vi "Zad1-2.vi"() -> ()   [LabVIEW 2015]
panel:
  in  "Losowanie":bool
  out "Numeric":dbl
  # "Losuj"
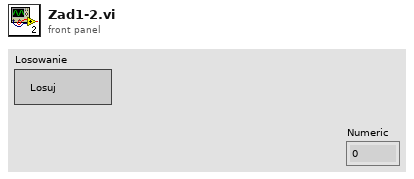
[diagram p1: front panel]
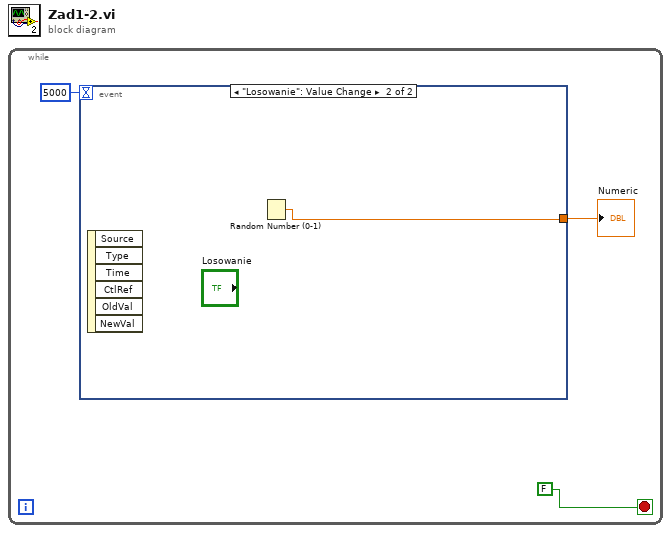
[diagram p0: block diagram]
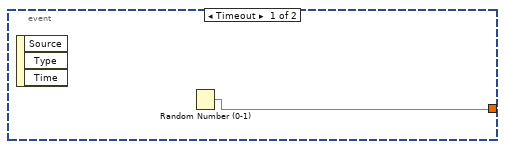
[diagram p2: hidden frame]
diagram:
  n1 = while {
    stop <- FALSE stop-if-true
    n2 = event shown="[1] \"Losowanie\": Value Change" {
      selector: _ -> [_ _]
      dyn-events: _ -> [_ _]
      timeout: 5000 -> [_ _]
      tunnel: [w4 w5] -> w1
      event Timeout {
        n3 = event-data() -> ()  [unwired: 1 in, 3 out]
        n4 = Random Number (0-1)() -> (number: 0 to 1=w4:dbl)
      }
      event "Losowanie": Value Change {
        n5 = event-data() -> ()  [unwired: 1 in, 6 out]
        n6 = Random Number (0-1)() -> (number: 0 to 1=w5:dbl)
      }
    }
    "Numeric" <- w1
  }
